vi "Controller - Fire LEDs change.vi"(8 "error in (no error)":errorcluster, 10 "LEDs status":T1, 11 "View Model":T2) -> (0 "error out":errorcluster, 3 "View Model":T2)   [LabVIEW 2017]
doc: "Generates user event when LED status is changed"
uses:
  View Model/Controls/View Model.ctl
  Configuration Database/Controls/Config Model.ctl
  Configuration Database/Controls/Config Commands.ctl
  Configuration Database/Controls/Congif Data.ctl
  View Model/Controls/Shared Model.ctl
  Error Handler/Controls/Error Model.ctl
  Error Handler/Controls/Error Data.ctl
  Error Handler/Controls/Error Type.ctl
  Controls/Car Wash Model.ctl
  Controls/Controller Overhead.ctl
  Controls/Vehicle Location.ctl
  Controls/Car Wash States.ctl
  Controls/CarWash CMD.ctl
  Views/Wash Display Console View/Controls/Car Wash Indicators.ctl
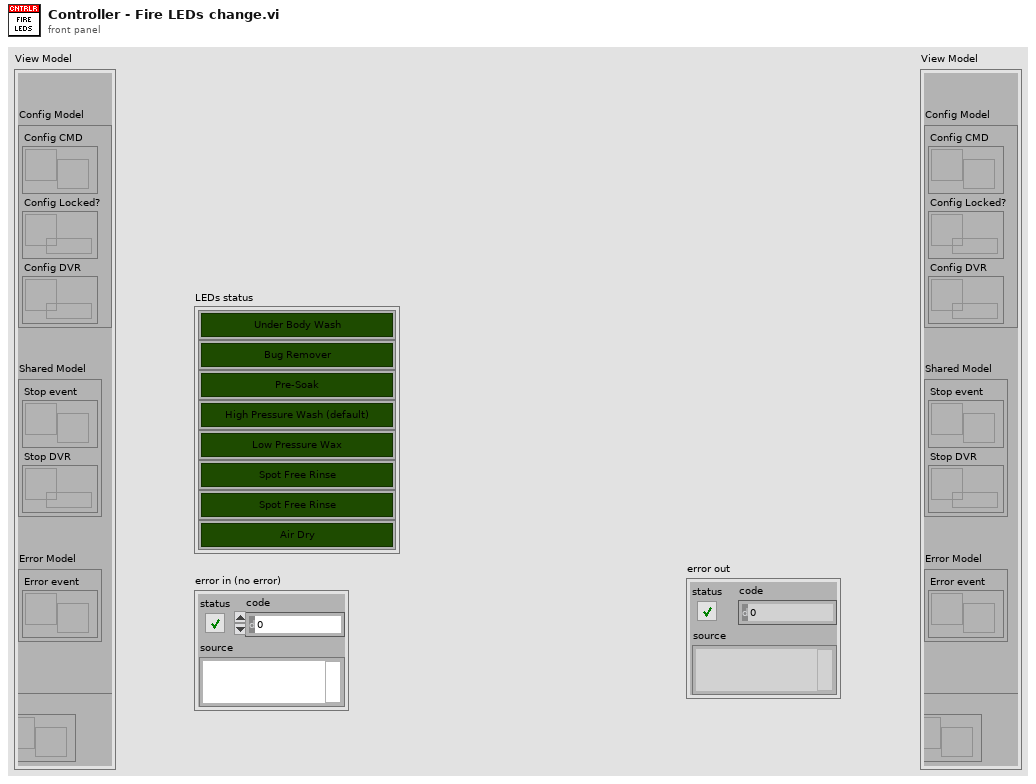
[diagram p1: front panel]
types:
  T1 = typedef "Car Wash Indicators.ctl" = cluster{"Under Body Wash":bool, "Bug Remover":bool, "Pre-Soak":bool, "High Pressure Wash":bool, "Low Pressure Wax":bool, "Spot Free Rinse":bool, "Tire Shine Foam":bool, "Air Dry":bool}
  T2 = typedef "View Model.ctl" = cluster{"Config Model":T3, "Shared Model":T4, "Error Model":T5, "Car Wash Model":T6}
  T3 = typedef "Config Model.ctl" = cluster{"Config CMD":refnum<user-event>, "Config Locked?":refnum<data-value>, "Config DVR":refnum<data-value>}
  T4 = typedef "Shared Model.ctl" = cluster{"Stop event":refnum<user-event>, "Stop DVR":refnum<data-value>}
  T5 = typedef "Error Model.ctl" = cluster{"Error event":refnum<user-event>}
  T6 = typedef "Car Wash Model.ctl" = cluster{"Out of Position Change":refnum<user-event>, "Wash Entry Change":refnum<user-event>, "Contr Overhead DVR":refnum<data-value>, "CarWash CMD":refnum<user-event>, "Location Change":refnum<user-event>, "Car Wash LEDs Change":refnum<user-event>}
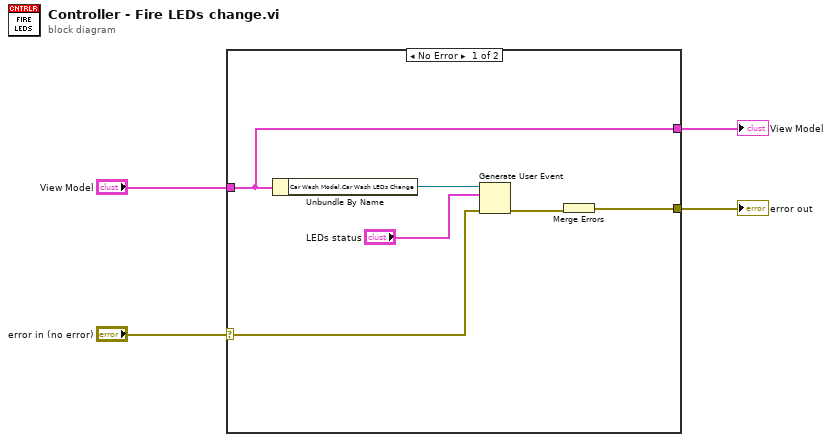
[diagram p0: block diagram]
diagram:
  n1 = case shown="No Error" "error in (no error)" {
    selector: "error in (no error)" -> [w9 w11]
    tunnel: "View Model" -> [w6 w12]
    tunnel: [w6 w12] -> w2
    tunnel: [w7 w11] -> w1
    frame No Error {
      n2 = Unbundle By Name(w6) -> ("Car Wash Model.Car Wash LEDs Change"=w10:refnum<user-event>)
      n3 = Generate User Event(user event=w10, event data cluster="LEDs status", error in=w9) -> (error out=w8:errorcluster)  [unwired: 1 in, 1 out]
      n4 = Merge Errors(w8) -> (w7:errorcluster)
    }
    frame Error {
    }
  }
  "View Model" <- w2
  "error out" <- w1
